vi "On Row Indent Accepted.vi"(4 "DragStart.Drag Indices":i32[](array[numeric]), 6 "DragStart.DragOver Same?":bool, 7 "Displayed Row":i32, 10 "TreeItem Indices (Displayed Items)":i32[](array[numeric]), 11 "TreeItems":T1[](array[typedef])) -> (1 "Allowed?":bool, 2 "indent":i32, 3 "Insertion index":i32)   [LabVIEW 2020, in "BetterDragAndDrop.lvlib" / "BetterTreeHandle.lvclass"]
uses:
  Classes/BetterTreeHandle/BetterTreeHandle.lvclass
  Classes/BetterTreeItem/SubVIs/TreeItem.ctl
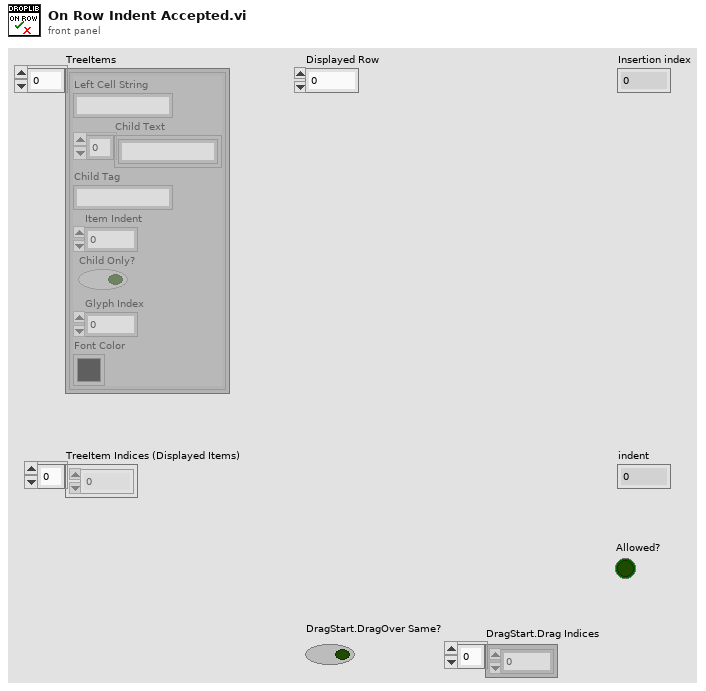
[diagram p1: front panel]
types:
  T1 = typedef "BetterDragAndDrop.lvlib/BetterTreeHandle.lvclass/TreeItem.ctl" = cluster{"Left Cell String":string, "Child Text":string[], "Child Tag":string, "Item Indent":i32, "Child Only?":bool, "Glyph Index":i32, "Font Color":u32}
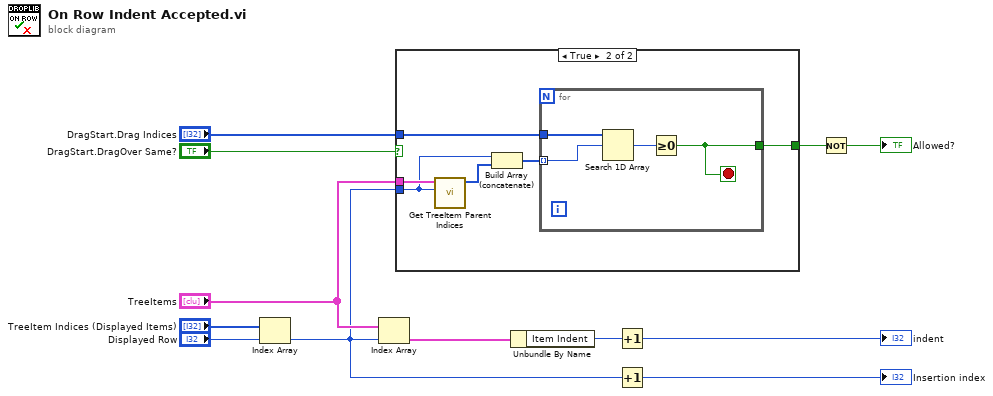
[diagram p0: block diagram]
diagram:
  n1 = Index Array(array="TreeItem Indices (Displayed Items)", index="Displayed Row") -> (element=w4:i32)
  n2 = Index Array(array="TreeItems", index=w4) -> (element=w8:T1)
  n3 = case shown="True" "DragStart.DragOver Same?" {
    tunnel: "DragStart.Drag Indices" -> [_ w17]
    tunnel: "TreeItems" -> [_ w18]
    tunnel: w4 -> [_ w15]
    tunnel: [_ w16] -> w6
    frame False {
    }
    frame True {
      n4 = call "Get TreeItem Parent Indices.vi"("TreeItem Index"=w15, "TreeItems"=w18) -> ("parent indices (incrementing)"=w14:i32[])  [unwired: 8 in, 1 out]
      n5 = Build Array (concatenate)(w15, w14) -> (w13:i32[])
      n6 = for {
        tunnel: w13 -> [w20] mode=indexing
        tunnel: w17 -> [w22]
        tunnel: [w19] -> w16
        stop <- w19 stop-if-true
        n7 = Search 1D Array(1D array=w22, element=w20) -> (index of element=w21:i32)  [unwired: 1 in]
        n8 = Greater Or Equal To 0?(x=w21) -> (x >= 0?=w19:bool)
      }
    }
  }
  n9 = Unbundle By Name(w8) -> ("Item Indent"=w10:i32)
  n10 = Increment(x=w10) -> (x+1=→"indent":i32)
  n11 = Increment(x=w4) -> (x+1=→"Insertion index":i32)
  n12 = Not(x=w6) -> (.not. x?=→"Allowed?":bool)
